vi "ShowCards.vi"(1 "Array 2":i16[](array[numeric])) -> (0 "Array":u16[](array[ring]))   [LabVIEW 2018]
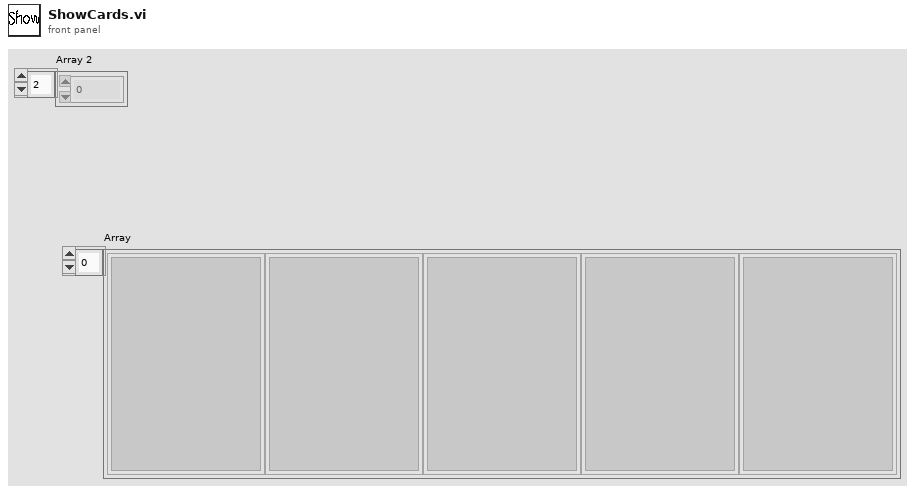
[diagram p1: front panel]
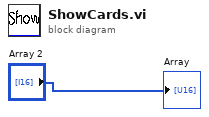
[diagram p0: block diagram]
diagram:
  "Array" <- "Array 2"
